vi "Angle Error.vi"(10 "Angle":dbl, 11 "Target Angle":dbl) -> (2 "Error":dbl)   [LabVIEW 2013]
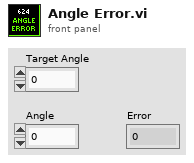
[diagram p1: front panel]
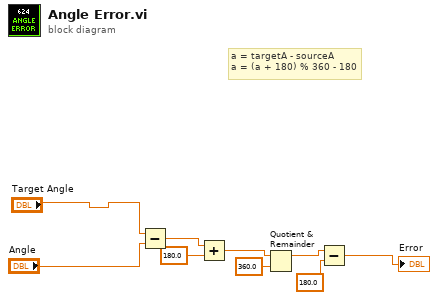
[diagram p0: block diagram]
diagram:
  # "a = targetA - sourceA\na = (a + 180) % 360 - 180"
  n1 = Subtract(x="Target Angle", y="Angle") -> (x-y=w8:dbl)
  n2 = Add(x=w8, y=180.0) -> (x+y=w5:dbl)
  n3 = Quotient & Remainder(x=w5, y=360.0) -> (x-y*floor(x/y)=w4:dbl)  [unwired: 1 out]
  n4 = Subtract(x=w4, y=180.0) -> (x-y=→"Error":dbl)
